vi "Get Units.vi"(8 "error in (no error)":errorcluster, 11 "Data in":refnum<class "Data.lvclass">) -> (0 "error out":errorcluster, 2 "Units out":refnum<class "Data.lvclass">, 3 "Data out":refnum<class "Data.lvclass">)   [LabVIEW 2015, in "MDSplus.lvlib" / "Data.lvclass"]
doc: "Return the units field. Return Empty if no units defined."
uses:
  <vilib>/MDSplus/Classes/Data_Class/Data.lvclass
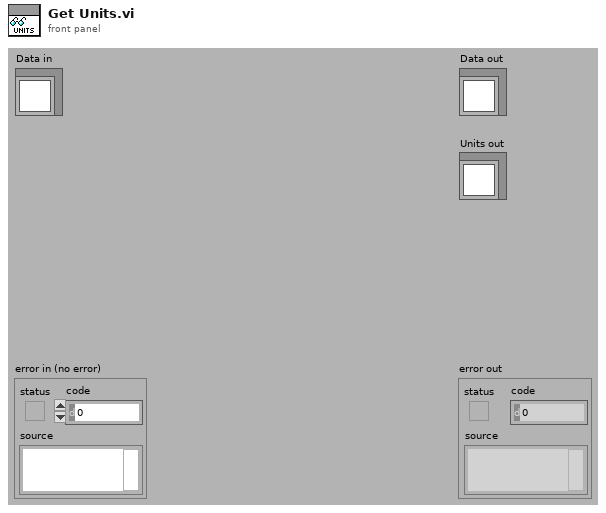
[diagram p1: front panel]
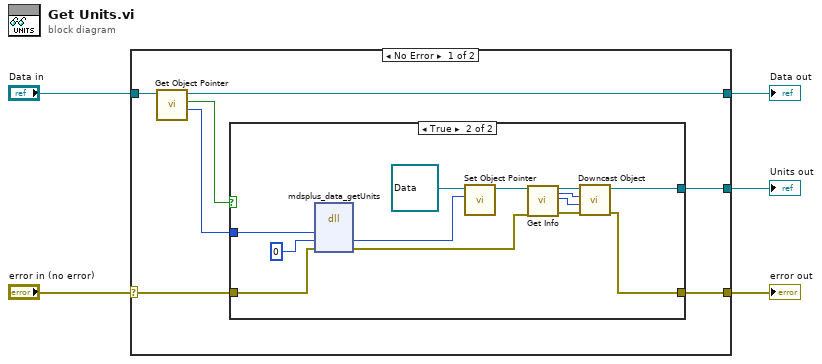
[diagram p0: block diagram]
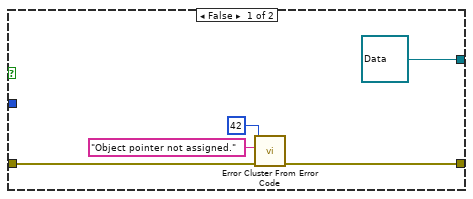
[diagram p2: hidden frame]
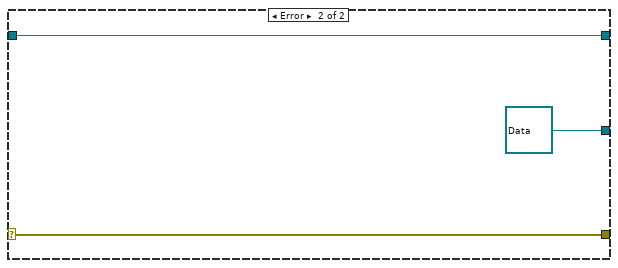
[diagram p3: hidden frame]
diagram:
  n1 = case shown="No Error" "error in (no error)" {
    selector: "error in (no error)" -> [w9 w33]
    tunnel: [w8 w33] -> w4
    tunnel: [w7 w32] -> w2
    tunnel: "Data in" -> [w12 w32]
    tunnel: [w6 refnum<class "Data.lvclass"> refnum ("Data out")] -> w1
    frame No Error {
      n2 = call-dynamic "Get Object Pointer.vi"("Data in"=w12) -> ("Object Pointer"=w10:i64, "Assigned object pointer?"=w11:bool, "Data out"=w7:refnum<class "Data.lvclass">)  [unwired: 8 in]
      n3 = case shown="True" w11 {
        tunnel: w10 -> [_ w30]
        tunnel: w9 -> [w15 w29]
        tunnel: [w14 w19] -> w8
        tunnel: [refnum<class "Data.lvclass"> refnum ("Data out") w18] -> w6
        frame False {
          n4 = call <vilib>:"Error Cluster From Error Code.vi"("error in (no error)"=w15, "error message (\"\")"="Object pointer not assigned." ("error message (\"\")"), "error code (0)"=42) -> ("error out"=w14:errorcluster)  [unwired: 6 in]
        }
        frame True {
          n5 = dll-call lib="MDSobjectsLVShr" fn="mdsplus_data_getUnits"("lvDataPtr"=w30, "lvDataPtrOut"=i64 0, "error"=w29) -> ("lvDataPtrOut"=w21:i64, "error"=w20:errorcluster)  [unwired: 5 in, 2 out]
          n6 = call-dynamic "Set Object Pointer.vi"("Object Pointer"=w21, "Data in"=refnum<class "Data.lvclass"> refnum ("Data.lvclass")) -> ("Data out"=w26:refnum<class "Data.lvclass">)  [unwired: 9 in]
          n7 = call-dynamic "Get Info.vi"("Data in"=w26, "error in (no error)"=w20) -> ("Data out"=w25:refnum<class "Data.lvclass">, "Class type out"=w24:u8, "Data type out"=w23:u8, "error out"=w22:errorcluster)  [unwired: 12 in, 2 out]
          n8 = call <vilib>:"Downcast Object.vi"("error in (no error)"=w22, "Data Type"=w23, "Class Type"=w24, "Data in"=w25) -> ("error out"=w19:errorcluster, "Data out"=w18:refnum<class "Data.lvclass">)  [unwired: 6 in]
        }
      }
    }
    frame Error {
    }
  }
  "error out" <- w4
  "Data out" <- w2
  "Units out" <- w1
